vi "setpointJSON.vi"(8 "Error in (no error)":errorcluster, 11 "Application ref in":refnum<vi>) -> (0 "Error out":errorcluster, 2 "JSON string":string, 3 "Application ref out":refnum<vi>)   [LabVIEW 2014]
uses:
  <userlib>/Nanonis Prog Interface V5/Nanonis Prog Interface.lvlib
panel:
  in  "setpoint":T1 {"Amplitude (m)" format="%#_6p"; "Z position (m)" format="%#_6p"; "Bias (V)" format="%_5p"; "Z Controller setpoint" format="%#_6p"}
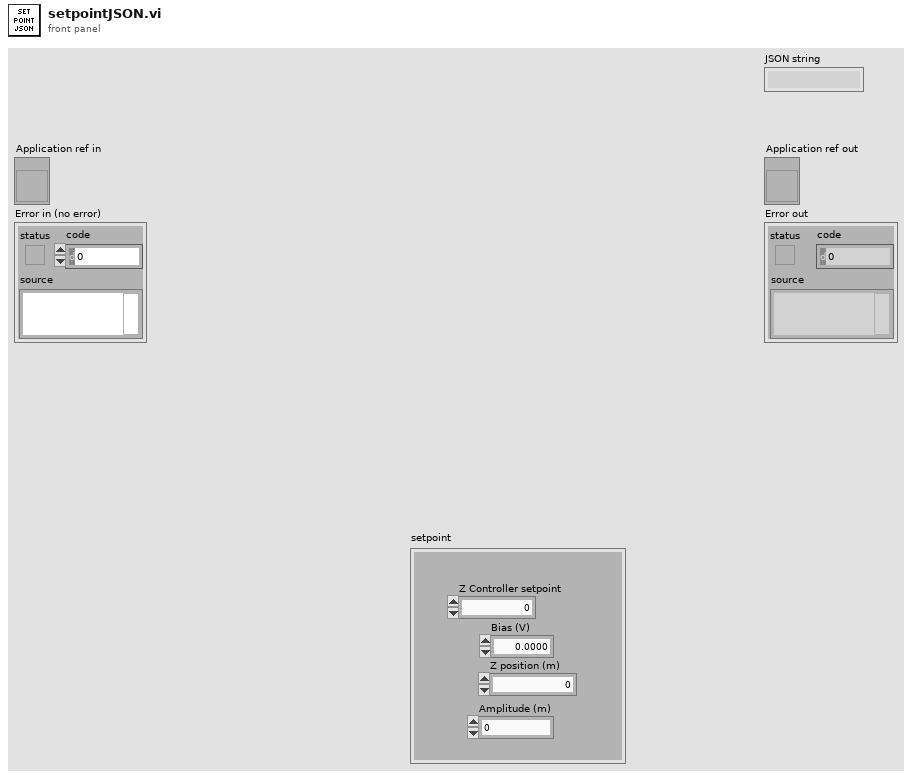
[diagram p1: front panel]
types:
  T1 = cluster{"Z Controller setpoint":sgl, "Bias (V)":sgl, "Z position (m)":sgl, "Amplitude (m)":sgl}
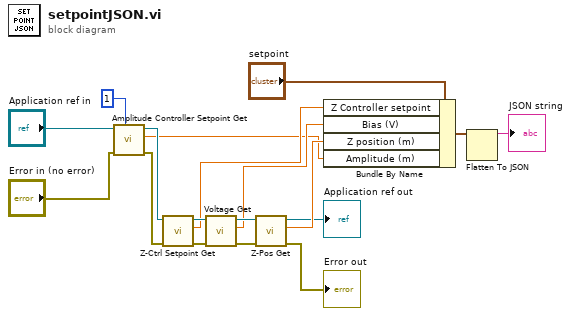
[diagram p0: block diagram]
diagram:
  n1 = call <userlib>:"Amplitude Controller Setpoint Get.vi"("Modulator index"=1, "Error in (no error)"="Error in (no error)", "Application ref in"="Application ref in") -> ("Error out"=w3:errorcluster, "Amplitude (m)"=w2:sgl, "Application ref out"=w5:refnum<vi>)  [unwired: 6 in]
  n2 = call <userlib>:"Z-Ctrl Setpoint Get.vi"("error in (no error)"=w3, "Application ref in"=w5) -> ("error out"=w18:errorcluster, "Z Controller setpoint"=w12:sgl, "Application ref out"=w17:refnum<vi>)  [unwired: 6 in]
  n3 = call <userlib>:"Voltage Get.vi"("error in (no error)"=w18, "Application ref in"=w17) -> ("error out"=w16:errorcluster, "Bias (V)"=w13:sgl, "Application ref out"=w15:refnum<vi>)  [unwired: 7 in]
  n4 = call <userlib>:"Z-Pos Get.vi"("error in (no error)"=w16, "Application ref in"=w15) -> ("error out"=→"Error out":errorcluster, "Z position (m)"=w11:sgl, "Application ref out"=→"Application ref out":refnum<vi>)  [unwired: 7 in]
  n5 = Bundle By Name(cluster="setpoint", "Z Controller setpoint"=w12, "Bias (V)"=w13, "Z position (m)"=w11, "Amplitude (m)"=w2) -> (w10:T1)
  n6 = Flatten To JSON(anything=w10) -> (JSON string=→"JSON string":string)  [unwired: 2 in, 1 out]
